vi "NoGoodFuture.vi"() -> ()   [LabVIEW 2019]
uses:
  <vilib>/userdefined/High Color/nirio_resource_hc.ctl
  <vilib>/myRIO/Instrument Drivers/Onboard IO/I2C/typedefs/I2C User Configuration.ctl
  <vilib>/myRIO/Instrument Drivers/Onboard IO/I2C/typedefs/I2C Transfer Rate.ctl
  <vilib>/myRIO/Instrument Drivers/Onboard IO/PWM/typedefs/PWM Reference.ctl
  <vilib>/myRIO/Common/Instrument Driver Framework/Utilities/typedefs/myRIO Generic Hardware Reference.ctl
  <vilib>/myRIO/Common/Instrument Driver Framework/Utilities/typedefs/Hardware Version Enum.ctl
  <vilib>/myRIO/Common/Instrument Driver Framework/Utilities/typedefs/myRIO v1.0 Reference.ctl
  <vilib>/myRIO/Common/Instrument Driver Framework/Utilities/typedefs/Generic FPGA Reference.ctl
  <vilib>/myRIO/Common/Instrument Driver Framework/myRIO v1.0/PWM/typedefs/PWM Channels Enum.ctl
  <vilib>/myRIO/Instrument Drivers/Onboard IO/PWM/typedefs/PWM Configuration.ctl
  <vilib>/myRIO/Instrument Drivers/Onboard IO/DIO/typedefs/DIO Reference.ctl
  <vilib>/myRIO/Common/Instrument Driver Framework/myRIO v1.0/DIO/typedefs/DIO Channels List.ctl
  <vilib>/myRIO/Common/Instrument Driver Framework/myRIO v1.0/DIO/typedefs/DIO Channels Enum.ctl
  <vilib>/myRIO/Common/Instrument Driver Framework/Utilities/vis/Is FPGA Ref Available.vi
  <vilib>/myRIO/Common/Instrument Driver Framework/myRIO v1.0/PWM/vis/myRIO v1.1 Open PWM.vi
  <vilib>/myRIO/Instrument Drivers/Onboard IO/PWM/vis/Set Duty Cycle and Frequency.vi
  <vilib>/myRIO/Common/Instrument Driver Framework/myRIO v1.0/DIO/vis/myRIO v1.1 Open DIO.vi
  <vilib>/myRIO/Common/Instrument Driver Framework/Utilities/vis/Validate Channels.vi
  <vilib>/myRIO/Common/Instrument Driver Framework/myRIO v1.0/PWM/vis/myRIO v1.0 Reserve PWM.vi
  <vilib>/myRIO/Common/Instrument Driver Framework/myRIO v1.0/DIO/vis/myRIO v1.0 Reserve DIO.vi
  <vilib>/myRIO/Common/Instrument Driver Framework/myRIO v1.0/I2C/vis/myRIO v1.0 Close I2C.vi
  <vilib>/myRIO/Common/Instrument Driver Framework/myRIO v1.0/UART/vis/myRIO v1.0 Close UART.vi
  <vilib>/myRIO/Common/Instrument Driver Framework/myRIO v1.0/PWM/vis/myRIO v1.0 Build MUX Configuration PWM.vi
  <vilib>/myRIO/Common/Instrument Driver Framework/myRIO v1.0/Resource Manager/vis/myRIO v1.0 Reserve Channel List.vi
  <vilib>/myRIO/Common/Instrument Driver Framework/myRIO v1.0/DIO/vis/myRIO v1.0 Build MUX Configuration DIO.vi
  <vilib>/myRIO/Common/Instrument Driver Framework/myRIO v1.0/I2C/vis/myRIO v1.0 Unreserve I2C.vi
  <vilib>/myRIO/Common/Instrument Driver Framework/myRIO v1.0/Resource Manager/vis/myRIO v1.0 Create Configuration List.vi
  <vilib>/myRIO/Common/Instrument Driver Framework/myRIO v1.0/Resource Manager/vis/myRIO v1.0 Reserve Channel.vi
  <vilib>/myRIO/Common/Instrument Driver Framework/myRIO v1.0/Resource Manager/vis/myRIO v1.0 Unreserve Channel.vi
  <vilib>/myRIO/Common/Instrument Driver Framework/myRIO v1.0/I2C/vis/myRIO v1.0 Build MUX Configuration I2C.vi
  <vilib>/myRIO/Common/Instrument Driver Framework/myRIO v1.0/Resource Manager/vis/myRIO v1.0 Unreserve Channel List.vi
  <vilib>/myRIO/Common/Instrument Driver Framework/myRIO v1.0/Resource Manager/vis/myRIO v1.0 Build Mutex Name.vi
  <vilib>/FPGAPlugInAG/myRIO-1900/niLvFpga_Open_myRIO-1900.vi
  <vilib>/rvi/interface/common/dynamic/niFpgaDynamicAddResources.vi
  <vilib>/Utility/error.llb/Error Cluster From Error Code.vi
  <vilib>/rvi/errors/niLvFpgaAdjustHostInterfaceError.vi
  <vilib>/myRIO/Common/Instrument Driver Framework/Utilities/vis/FPGA Ref Manager.vi
  <vilib>/myRIO/Common/Instrument Driver Framework/Utilities/vis/Ref Counter.vi
  <vilib>/FPGAPlugInAG/Dynamic/niLvFpga_Run_Dynamic.vi
  <vilib>/Utility/VariantDataType/GetNumericInfo.vi
  <vilib>/myRIO/Common/Instrument Driver Framework/myRIO v1.0/myRIO v1.1 Open.vi
  <vilib>/myRIO/Common/Instrument Driver Framework/Utilities/vis/IO Manager.vi
  <vilib>/myRIO/Common/Instrument Driver Framework/Utilities/vis/Configuration Manager.vi
  <vilib>/myRIO/Common/Instrument Driver Framework/myRIO v1.0/Resource Manager/vis/myRIO v1.0 Configure IO.vi
  <vilib>/myRIO/Common/Instrument Driver Framework/myRIO v1.0/myRIO v1.0 Close.vi
  <vilib>/myRIO/Common/Instrument Driver Framework/myRIO v1.0/PWM/vis/myRIO v1.0 Write PWM.vi
  <vilib>/myRIO/Common/Instrument Driver Framework/myRIO v1.0/DIO/vis/myRIO v1.0 Write DIO.vi
  <vilib>/myRIO/Common/Instrument Driver Framework/myRIO v1.0/I2C/vis/myRIO v1.0 Configure I2C.vi
  <vilib>/myRIO/Common/Instrument Driver Framework/myRIO v1.0/I2C/vis/myRIO v1.0 Write I2C.vi
  <vilib>/myRIO/Common/Instrument Driver Framework/myRIO v1.0/I2C/vis/myRIO v1.0 Read I2C.vi
  <vilib>/myRIO/Common/Instrument Driver Framework/myRIO v1.0/I2C/vis/myRIO v1.0 Shutdown I2C.vi
  <vilib>/FPGAPlugInAG/Dynamic/niLvFpga_Abort_Dynamic.vi
  <vilib>/myRIO/Common/Instrument Driver Framework/myRIO v1.0/myRIO v1.0 Reset FPGA.vi
  <vilib>/myRIO/Common/Instrument Driver Framework/myRIO v1.0/IRQ/vis/myRIO v1.0 IRQ Info FGV.vi
  <vilib>/myRIO/Common/Instrument Driver Framework/myRIO v1.0/IRQ/vis/myRIO v1.0 Timer IRQ Info FGV.vi
  <vilib>/myRIO/Common/Instrument Driver Framework/myRIO v1.0/IRQ/vis/myRIO v1.0 ISR Agent.vi
  <vilib>/myRIO/Instrument Drivers/Utilities/vis/Reset Index.vi
  <vilib>/myRIO/Common/Instrument Driver Framework/myRIO v1.0/Resource Manager/vis/myRIO v1.0 Block Write Resource Manager.vi
  <vilib>/FPGAPlugInAG/Dynamic/niLvFpga_Close_Dynamic.vi
  <vilib>/rvi/interface/nirviOpenFPGA/nirviOpenFPGA.xnode
  CustomFPGA.lvbitx
  <vilib>/rvi/interface/nirviReadWriteControl/nirviReadWriteControl.xnode
  <vilib>/rvi/interface/nirviMethod/nirviMethod.xnode
  <vilib>/myRIO/Express VI/Onboard IO/PWM/PWM Express VI.xnode
  <vilib>/myRIO/Instrument Drivers/Onboard IO/PWM/vis/myRIO PWM Open.xnode
  <vilib>/myRIO/Express VI/Onboard IO/DO/DO Express VI.xnode
  <vilib>/myRIO/Instrument Drivers/Onboard IO/DIO/vis/myRIO DIO Open.xnode
  <vilib>/rvi/interface/nirviCloseFPGA/nirviCloseFPGA.xnode
  <vilib>/myRIO/Instrument Drivers/Utilities/Utilities.lvlib
  NiFpgaLv.dll
  <vilib>/rvi/interface/Simulation/niFpgaSimulationCallBeginRW.vi
  <vilib>/myRIO/Instrument Drivers/Onboard IO/I2C/I2C.lvlib
  <vilib>/myRIO/Instrument Drivers/Onboard IO/DIO/DIO.lvlib
  <vilib>/myRIO/Instrument Drivers/Onboard IO/PWM/PWM.lvlib
panel:
  in  "stop":bool
  out "Acc":dbl[](array[numeric])
  out "Gyro":dbl[](array[numeric])
  out "E-Stop":bool
  out "Velocity (Counts/Interval)":i32
  out "Acceleration (Counts/Interval)":i32
  out "Position (Counts)":i32
  out "Hall Period":u32
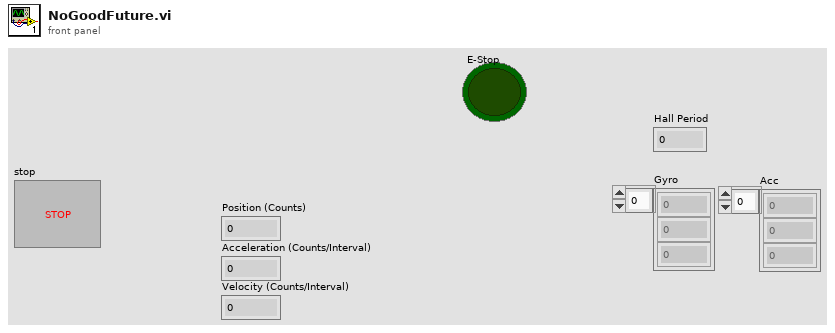
[diagram p1: front panel]
types:
  T1 = typedef "nirio_resource_hc.ctl" = tag
  T2 = typedef "PWM.lvlib/PWM Reference.ctl" = cluster{"myRIO Reference":T3, "PWM Channels Enum":T7, "PWM Configuration":T8}
  T3 = typedef "myRIO Generic Hardware Reference.ctl" = cluster{"myRIO Model":T4, "myRIO Hardware Reference":T5}
  T4 = typedef "Hardware Version Enum.ctl" = enum16{"Unknown", "myRIO-1900", "myRIO-1950", "roboRIO", "NI ELVIS RIO CM", "ELVIS III"}
  T5 = typedef "myRIO v1.0 Reference.ctl" = cluster{"Generic FPGA Reference":T6, "Allow multiple opens":bool}
  T6 = typedef "Generic FPGA Reference.ctl" = refnum<k20>
  T7 = typedef "PWM Channels Enum.ctl" = enum16{"Not Connected", "C/PWM0", "C/PWM1", "A/PWM0", "A/PWM1", "A/PWM2", "A/PWM3", "A/PWM4", "A/PWM5", "A/PWM6", "A/PWM7", "A/PWM8", "A/PWM9", "A/PWM10", "A/PWM11", "A/PWM12", "A/PWM13", "A/PWM14", "A/PWM15", "A/PWM16", "A/PWM17", "A/PWM18", "A/PWM19", "B/PWM0", "B/PWM1", "B/PWM2", "B/PWM3", "B/PWM4", "B/PWM5", "B/PWM6", "B/PWM7", "B/PWM8", "B/PWM9", "B/PWM10", "B/PWM11", "B/PWM12", "B/PWM13", "B/PWM14", "B/PWM15", "B/PWM16", "B/PWM17", "B/PWM18", "B/PWM19", "PWM/PWM0", "PWM/PWM1", "PWM/PWM2", "PWM/PWM3", "PWM/PWM4", "PWM/PWM5", "PWM/PWM6", "PWM/PWM7", "PWM/PWM8", "PWM/PWM9"}
  T8 = typedef "PWM.lvlib/PWM Configuration.ctl" = cluster{"Frequency":dbl, "Duty Cycle":dbl}
  T9 = typedef "DIO.lvlib/DIO Reference.ctl" = cluster{"myRIO Reference":T3, "DIO Channels List":T10}
  T10 = typedef "DIO Channels List.ctl" = T11[]
  T11 = typedef "DIO Channels Enum.ctl" = enum16{"Not Connected", "C/DIO0", "C/DIO1", "C/DIO2", "C/DIO3", "C/DIO4", "C/DIO5", "C/DIO6", "C/DIO7", "A/DIO0", "A/DIO1", "A/DIO2", "A/DIO3", "A/DIO4", "A/DIO5", "A/DIO6", "A/DIO7", "A/DIO8", "A/DIO9", "A/DIO10", "A/DIO11", "A/DIO12", "A/DIO13", "A/DIO14", "A/DIO15", "A/DIO16", "A/DIO17", "A/DIO18", "A/DIO19", "B/DIO0", "B/DIO1", "B/DIO2", "B/DIO3", "B/DIO4", "B/DIO5", "B/DIO6", "B/DIO7", "B/DIO8", "B/DIO9", "B/DIO10", "B/DIO11", "B/DIO12", "B/DIO13", "B/DIO14", "B/DIO15", "B/DIO16", "B/DIO17", "B/DIO18", "B/DIO19", "LED0", "LED1", "LED2", "LED3", "Button0", "DIO/DIO0", "DIO/DIO1", "DIO/DIO2", "DIO/DIO3", "DIO/DIO4", "DIO/DIO5", "DIO/DIO6", "DIO/DIO7", "DIO/DIO8", "DIO/DIO9", "SPI/CS0", "SPI/CS1", "SPI/CS2", "SPI/CS3", "LED RADIO (Green)", "LED RADIO (Red)", "LED COMM (Green)", "LED COMM (Red)", "LED MODE (Green)", "LED MODE (Red)"}
  T12 = typedef "I2C.lvlib/I2C User Configuration.ctl" = cluster{"I2C Transfer Rate":T13}
  T13 = typedef "I2C.lvlib/I2C Transfer Rate.ctl" = enum16{"Standard mode (100 kbps)", "Fast mode (400 kbps)"}
  T14 = typedef "I2C.lvlib/I2C Reference.ctl" = cluster{"myRIO Reference":T3, "I2C Channels Enum":T15, "I2C Configuration":T16}
  T15 = typedef "I2C Channels Enum.ctl" = enum16{"Not Connected", "A/I2C", "B/I2C", "I2C/I2C"}
  T16 = typedef "I2C.lvlib/I2C Configuration.ctl" = cluster{"I2C Transfer Rate":T13}
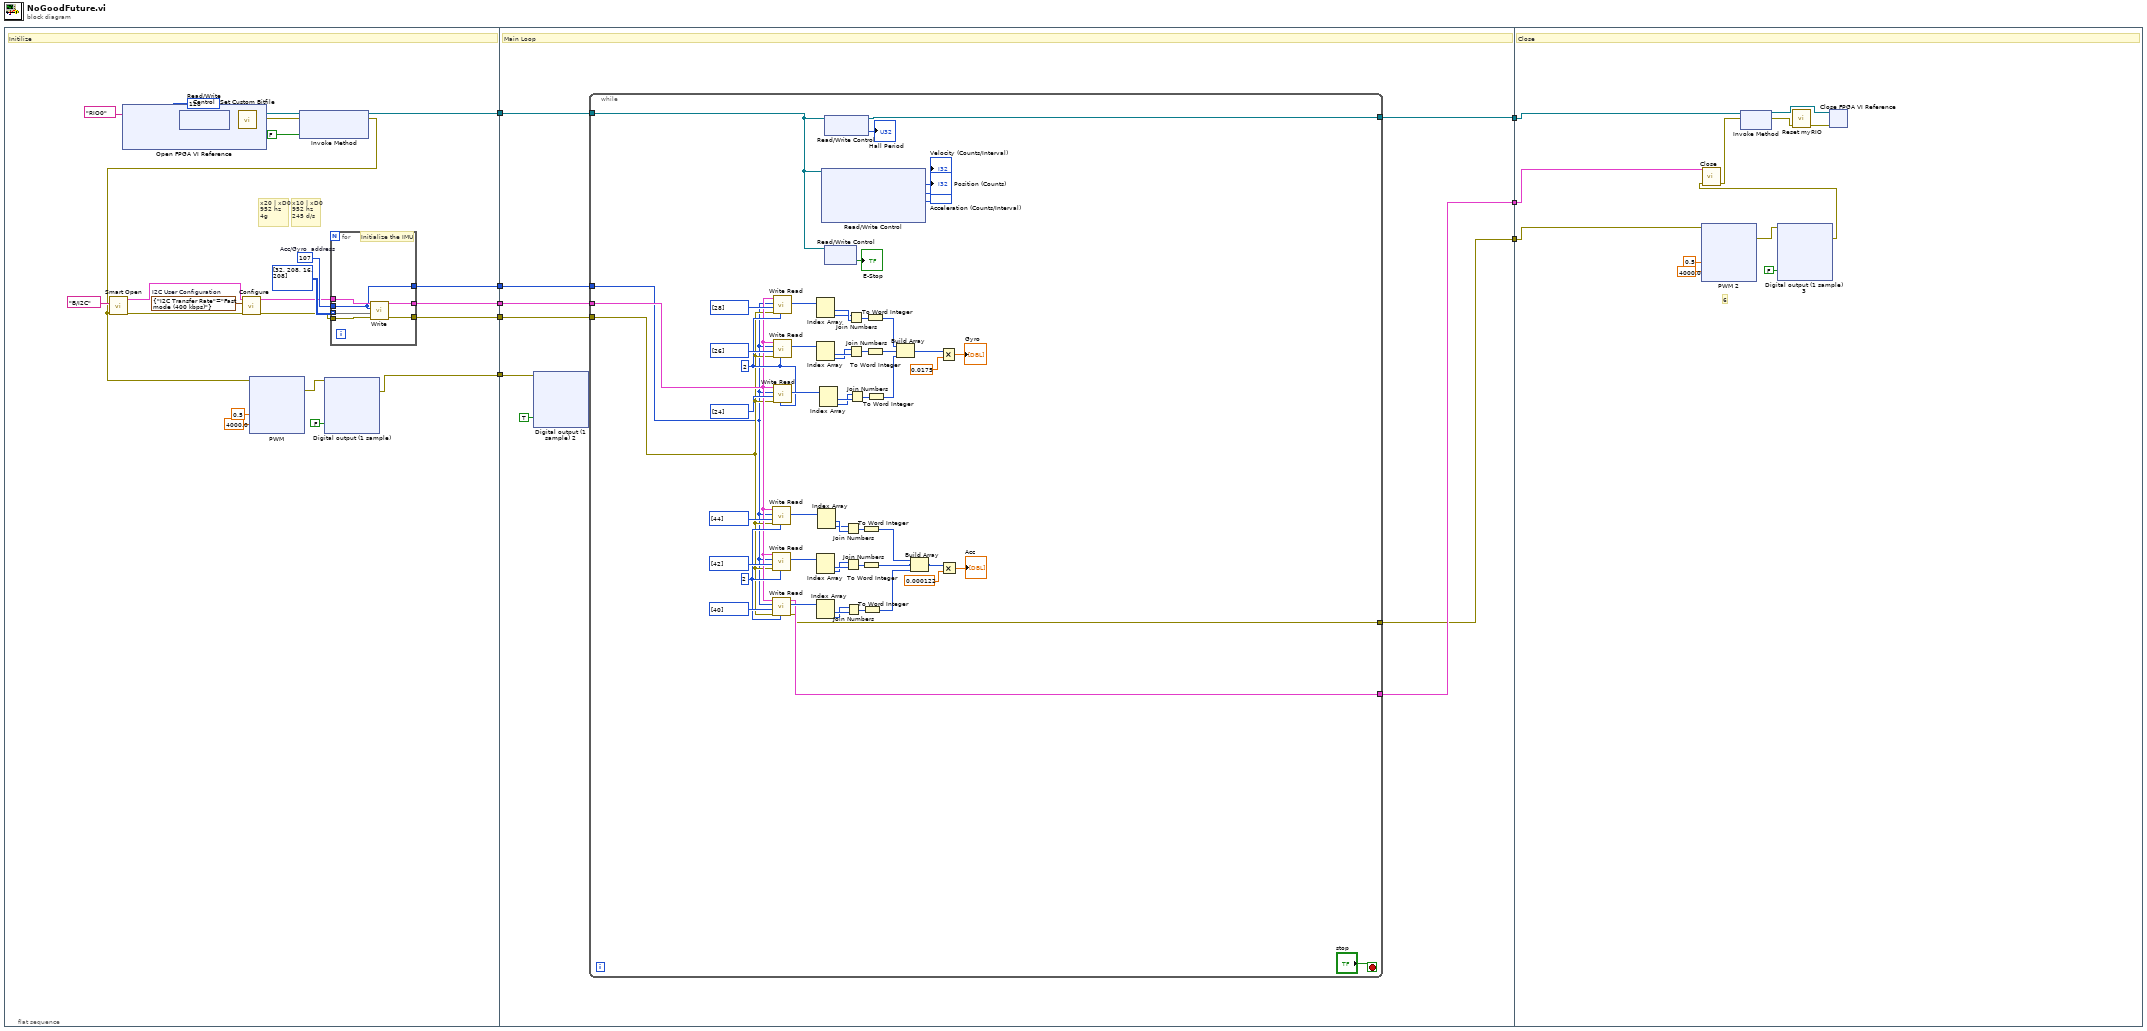
[diagram p0: block diagram]
diagram:
  n1 = flat-sequence {
    tunnel: [w13] -> w8
    tunnel: [w12] -> w7
    tunnel: [w11] -> w6
    tunnel: [w10] -> w5
    tunnel: [w9] -> w4
    tunnel: w8 -> [w120]
    tunnel: w7 -> [w119]
    tunnel: w6 -> [w118]
    tunnel: w5 -> [w117]
    tunnel: w4 -> [w116]
    tunnel: [w114] -> w3
    tunnel: [w113] -> w2
    tunnel: [w112] -> w1
    tunnel: w3 -> [w216]
    tunnel: w2 -> [w217]
    tunnel: w1 -> [w213]
    frame #0 {
      w22 = u8 107  # Acc/Gyro  address
      w24 = T12 {"I2C Transfer Rate"=enum."Fast mode (400 kbps)"}  # I2C User Configuration
      # "x20 | xD0\n952 hz\n4g"
      # "x10 | xD0\n952 hz\n245 d/s"
      # "Initilize"
      n2 = xnode "Open FPGA VI Reference"("resource name"=T1 "RIO0" ("Resource name")) -> ("FPGA VI Reference Out"=w28:refnum<k20>, "error out"=w27:errorcluster)  [unwired: 1 in]
      n3 = xnode "Read/Write Control"("FPGA VI Reference In"=w28, "error in"=w27, "SYS.SELECTB"=u8 128) -> ("FPGA VI Reference Out"=w32:refnum<k20>, "error out"=w31:errorcluster)
      n4 = call <vilib>:"Set Custom Bitfile.vi"("error in (no error)"=w31, "Custom FPGA Reference In"=w32) -> ("error out"=w33:errorcluster, "Custom FPGA Reference Out"=w35:refnum<k20>)  [unwired: 8 in]
      n5 = xnode "Invoke Method"("FPGA VI Reference In"=w35, "error in"=w33, "Wait Until Done (F)"=FALSE) -> ("FPGA VI Reference Out"=w13:refnum<k20>, "error out"=w14:errorcluster)
      n6 = call <vilib>:"Smart Open.vi"("error in (no error)"=w14, "Channel Name"=tag "B/I2C" ("I2C I/O")) -> ("error out"=w26:errorcluster, "I2C Ref Out"=w25:T14)  [unwired: 8 in]
      n7 = call <vilib>:"Configure.vi"("error in (no error)"=w26, "I2C User Configuration"=w24, "I2C Ref In"=w25) -> ("error out"=w20:errorcluster, "I2C Ref Out"=w21:T14)  [unwired: 7 in]
      n8 = xnode "PWM"("Duty Cycle"=0.5, "Frequency [Hz]"=4000.0, "error in (no error)"=w14) -> ("error out"=w18:errorcluster)
      n9 = xnode "Digital output (1 sample)"("B/DIO13 (Pin 26)"=FALSE ("B/DIO1 (Pin 13)"), "error in (no error)"=w18) -> ("error out"=w9:errorcluster)
      n10 = for {
        tunnel: [w110] -> w10
        tunnel: [w111] -> w11
        tunnel: u8[][] [[32, 208], [16, 208]] ("Bytes to Write") -> [w109] mode=indexing
        tunnel: w22 -> [w106]
        tunnel: w21 -> [w108]
        tunnel: w20 -> [w107]
        tunnel: [w106] -> w12
        # "Initialize the IMU"
        n11 = call <vilib>:"Write.vi"("error in (no error)"=w107, "Bytes to Write"=w109, "Slave Address (7-bit)"=w106, "I2C Ref In"=w108) -> ("error out"=w110:errorcluster, "I2C Ref Out"=w111:T14)  [unwired: 6 in]
      }
    }
    frame #1 {
      # "Main Loop"
      n12 = xnode "Digital output (1 sample) 2"("B/DIO13 (Pin 26)"=TRUE, "error in (no error)"=w116) -> ()  [unwired: 1 out]
      n13 = while {
        tunnel: w120 -> [w212]
        tunnel: w119 -> [w175]
        tunnel: w118 -> [w177]
        tunnel: w117 -> [w176]
        tunnel: [w158] -> w114
        tunnel: [w157] -> w113
        tunnel: [w156] -> w112
        stop <- "stop" stop-if-true
        w180 = u32 2 ("Byte Count")
        w196 = u32 2 ("Byte Count")
        n14 = call <vilib>:"Write Read.vi"("Byte Count"=w196, "error in (no error)"=w176, "Bytes to Write"=u8[] [44], "Slave Address (7-bit)"=w175, "I2C Ref In"=w177) -> ("Bytes Read"=w204:u8[])  [unwired: 3 in, 2 out]
        n15 = call <vilib>:"Write Read.vi"("Byte Count"=w196, "error in (no error)"=w176, "Bytes to Write"=u8[] [42], "Slave Address (7-bit)"=w175, "I2C Ref In"=w177) -> ("Bytes Read"=w206:u8[])  [unwired: 3 in, 2 out]
        n16 = call <vilib>:"Write Read.vi"("Byte Count"=w196, "error in (no error)"=w176, "Bytes to Write"=u8[] [40], "Slave Address (7-bit)"=w175, "I2C Ref In"=w177) -> ("error out"=w156:errorcluster, "Bytes Read"=w208:u8[], "I2C Ref Out"=w158:T14)  [unwired: 3 in]
        n17 = call <vilib>:"Write Read.vi"("Byte Count"=w180, "error in (no error)"=w176, "Bytes to Write"=u8[] [28], "Slave Address (7-bit)"=w175, "I2C Ref In"=w177) -> ("Bytes Read"=w188:u8[])  [unwired: 3 in, 2 out]
        n18 = call <vilib>:"Write Read.vi"("Byte Count"=w180, "error in (no error)"=w176, "Bytes to Write"=u8[] [26], "Slave Address (7-bit)"=w175, "I2C Ref In"=w177) -> ("Bytes Read"=w190:u8[])  [unwired: 3 in, 2 out]
        n19 = call <vilib>:"Write Read.vi"("Byte Count"=w180, "error in (no error)"=w176, "Bytes to Write"=u8[] [24], "Slave Address (7-bit)"=w175, "I2C Ref In"=w177) -> ("Bytes Read"=w192:u8[])  [unwired: 3 in, 2 out]
        n20 = Index Array "Index Array"(array=w188) -> (element #1=w186:u8, element #2=w185:u8)  [unwired: 2 in]
        n21 = Index Array "Index Array"(array=w190) -> (element #1=w184:u8, element #2=w183:u8)  [unwired: 2 in]
        n22 = Index Array "Index Array"(array=w206) -> (element #1=w200:u8, element #2=w199:u8)  [unwired: 2 in]
        n23 = Index Array "Index Array"(array=w208) -> (element #1=w198:u8, element #2=w197:u8)  [unwired: 2 in]
        n24 = Index Array "Index Array"(array=w204) -> (element #1=w202:u8, element #2=w201:u8)  [unwired: 2 in]
        n25 = Index Array "Index Array"(array=w192) -> (element #1=w182:u8, element #2=w181:u8)  [unwired: 2 in]
        n26 = xnode "Read/Write Control"("FPGA VI Reference In"=w212) -> ("Position (Counts)"=→"Position (Counts)":i32, "Acceleration (Counts/Interval)"=→"Acceleration (Counts/Interval)":i32, "Velocity (Counts/Interval)"=→"Velocity (Counts/Interval)":i32)  [unwired: 3 in, 2 out]
        n27 = xnode "Read/Write Control"("FPGA VI Reference In"=w212) -> ("FPGA VI Reference Out"=w157:refnum<k20>, "Hall Period"=→"Hall Period":u32)  [unwired: 1 in, 1 out]
        n28 = xnode "Read/Write Control"("FPGA VI Reference In"=w212) -> ("E-Stop"=→"E-Stop":bool)  [unwired: 1 in, 2 out]
        n29 = Join Numbers(hi=w201, lo=w202) -> ((hi.lo)=w211:u16)
        n30 = Join Numbers(hi=w199, lo=w200) -> ((hi.lo)=w210:u16)
        n31 = Join Numbers(hi=w197, lo=w198) -> ((hi.lo)=w209:u16)
        n32 = Join Numbers(hi=w185, lo=w186) -> ((hi.lo)=w195:u16)
        n33 = Join Numbers(hi=w183, lo=w184) -> ((hi.lo)=w194:u16)
        n34 = Join Numbers(hi=w181, lo=w182) -> ((hi.lo)=w193:u16)
        n35 = To Word Integer(number=w211) -> (16bit integer=w170:i16)
        n36 = To Word Integer(number=w210) -> (16bit integer=w169:i16)
        n37 = To Word Integer(number=w209) -> (16bit integer=w168:i16)
        n38 = To Word Integer(number=w195) -> (16bit integer=w174:i16)
        n39 = To Word Integer(number=w194) -> (16bit integer=w173:i16)
        n40 = To Word Integer(number=w193) -> (16bit integer=w172:i16)
        n41 = Build Array(w174, w173, w172) -> (w171:i16[])
        n42 = Build Array(w170, w169, w168) -> (w167:i16[])
        n43 = Multiply(x=w171, y=0.0175) -> (x*y=→"Gyro":dbl[])
        n44 = Multiply(x=w167, y=0.000122) -> (x*y=→"Acc":dbl[])
      }
    }
    frame #2 {
      # "6"
      # "Close"
      n45 = xnode "PWM 2"("Duty Cycle"=0.5, "Frequency [Hz]"=4000.0, "error in (no error)"=w213) -> ("error out"=w222:errorcluster)
      n46 = xnode "Digital output (1 sample) 3"("B/DIO13 (Pin 26)"=FALSE ("B/DIO1 (Pin 13)"), "error in (no error)"=w222) -> ("error out"=w215:errorcluster)
      n47 = call <vilib>:"Close.vi"("error in (no error)"=w215, "I2C Ref In"=w216) -> ("error out"=w214:errorcluster)  [unwired: 9 in]
      n48 = xnode "Invoke Method"("FPGA VI Reference In"=w217, "error in"=w214) -> ("FPGA VI Reference Out"=w221:refnum<k20>, "error out"=w219:errorcluster)
      n49 = call <vilib>:"Reset myRIO.vi"("error in (no error)"=w219) -> ("error out"=w220:errorcluster)  [unwired: 10 in]
      n50 = xnode "Close FPGA VI Reference"("FPGA VI Reference In"=w221, "error in"=w220) -> ()  [unwired: 1 out]
    }
  }
